vi "Module_ENG_SocketServer.vi"(8 "error in (no error)":errorcluster, 9 "Module ID (-1: Do not Address)":i32=-1, 10 "Wait on Module(s) (\"\": none)":string) -> (0 "error out":errorcluster)   [LabVIEW 2019, in "Module_ENG_SocketServer.lvclass"]
doc: "created using\nJSMA Module Template - ENGINE Class 0.2.1.12\nRob Humfeld - Jet Engineering\nCopyright (c) 2020, Jet Engineering"
uses:
  Module_ENG_SocketServer.lvclass
  <userlib>/Jet Engineering/JSMA/Libraries/jModule Class/Typedefs/jModule_TimerConfig STYP.ctl
  <userlib>/Jet Engineering/JSMA/Libraries/jModule Class/Typedefs/jModule_TimerType STYP.ctl
  Private/Module_ENG_SocketServer_jMsgTxList STYP.ctl
  <userlib>/Jet Engineering/JSMA/Libraries/jMsg_CORE/jMsg_JSMA_ModuleOnline/jMsg_JSMA_ModuleOnline.lvclass
  C:/Program Files/National Instruments/LabVIEW 2019/user.lib/Jet Engineering/JSMA/Libraries/jMsg Class/jMsg.lvclass
  Private/Module_ENG_SocketServer_jMsgRxList STYP.ctl
  <userlib>/Jet Engineering/JSMA/Libraries/jMsg_CORE/jMsg_JSMA_ApplicationShutdown/jMsg_JSMA_ApplicationShutdown.lvclass
  C:/Program Files/National Instruments/LabVIEW 2019/user.lib/Jet Engineering/JSMA/Libraries/jModule Class/jModule.lvclass
  Private/Module_ENG_SocketServer_LocalData STYP.ctl
  Private/Module_ENG_SocketServer_EngineStatus STYP.ctl
  <userlib>/Jet Engineering/JET_QSM/Code/Private/JET_QSM_InvalidOption STYP.ctl
  <userlib>/Jet Engineering/JSMA/Libraries/jModule Class/jModule.lvclass/jModule.ctl
  Module_ENG_SocketServer.lvclass/Module_ENG_SocketServer.ctl
  <userlib>/Jet Engineering/JET_QSM/Code/Private/JET_QSM - Add State [String API].vi
  <userlib>/Jet Engineering/JSMA/Libraries/jModule Class/Read Timeout Configuration.vi
  <userlib>/Jet Engineering/JET_QSM/Code/Private/JET_QSM - Add State to Front [String API].vi
  <vilib>/Utility/error.llb/Trim Whitespace.vi
  <vilib>/Utility/error.llb/Error Cluster From Error Code.vi
  <userlib>/Jet Engineering/JSMA/Libraries/jModule Class/jModule.lvclass
panel:
  out "Timer Configuration":T1 {"Expiration Time" format="%<%.3X>T"}
  out "jModule Name":string
  out "iter":i32
  out "Latency, sec.":dbl
  out "RxTime":timestamp format="%<%H:%M:%S%3u>T"
  out "Last Rx Message":string
  out "Recent states before Error (with tick counts)":string
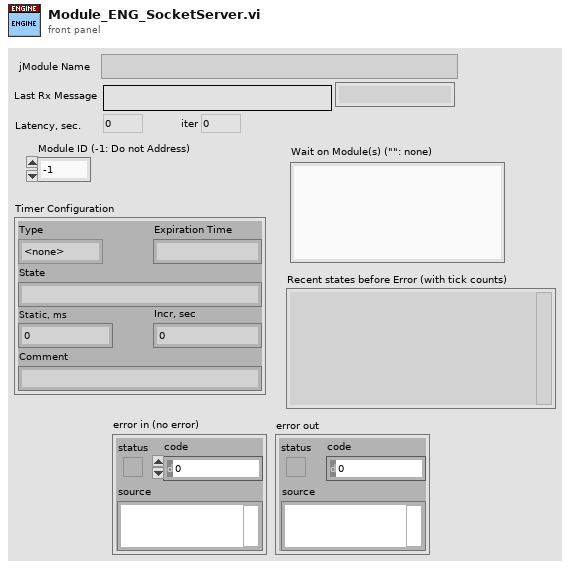
[diagram p1: front panel]
types:
  T1 = typedef "JSMA API.lvlib/jModule.lvclass/jModule_TimerConfig STYP.ctl" = cluster{"Type":T2, "Expiration Time":timestamp, "State":string, "Static, ms":i32, "Incr, sec":dbl, "Comment":string}
  T2 = typedef "JSMA API.lvlib/jModule.lvclass/jModule_TimerType STYP.ctl" = enum16{"<none>", "Static", "Countdown", "Periodic"}
  T3 = typedef "JET_QSM_InvalidOption STYP.ctl" = enum16{"Ignore", "Dialog", "Error"}
  T4 = typedef "Module_ENG_SocketServer.lvclass/Module_ENG_SocketServer_LocalData STYP.ctl" = cluster{"VI":cluster{"error":errorcluster, "isExiting?":bool}, "EngineStatus":T5}
  T5 = typedef "Module_ENG_SocketServer.lvclass/Module_ENG_SocketServer_EngineStatus STYP.ctl" = cluster{"<placeholder>":bool}
  T6 = typedef "Module_ENG_SocketServer.lvclass/Module_ENG_SocketServer_jMsgRxList STYP.ctl" = cluster{"<placeholder>":refnum<class "jMsg_JSMA_ApplicationShutdown.lvclass">}
  T7 = typedef "Module_ENG_SocketServer.lvclass/Module_ENG_SocketServer_jMsgTxList STYP.ctl" = cluster{"<placeholder>":refnum<class "jMsg_JSMA_ModuleOnline.lvclass">}
  T8 = typedef "JET_QSM_Refnum STYP.ctl" = cluster{"state":cluster{"queue":refnum<queue>, "idle":string, "error":string, "STOP":string}, "debug":cluster{"enabled?":bool, "queue":refnum<queue>}, "Invalid.option":T3, "QSM.Name":string}
  T9 = typedef "JET_QSM_Element STYP.ctl" = cluster{"state":string, "data":variant, "comment":string}
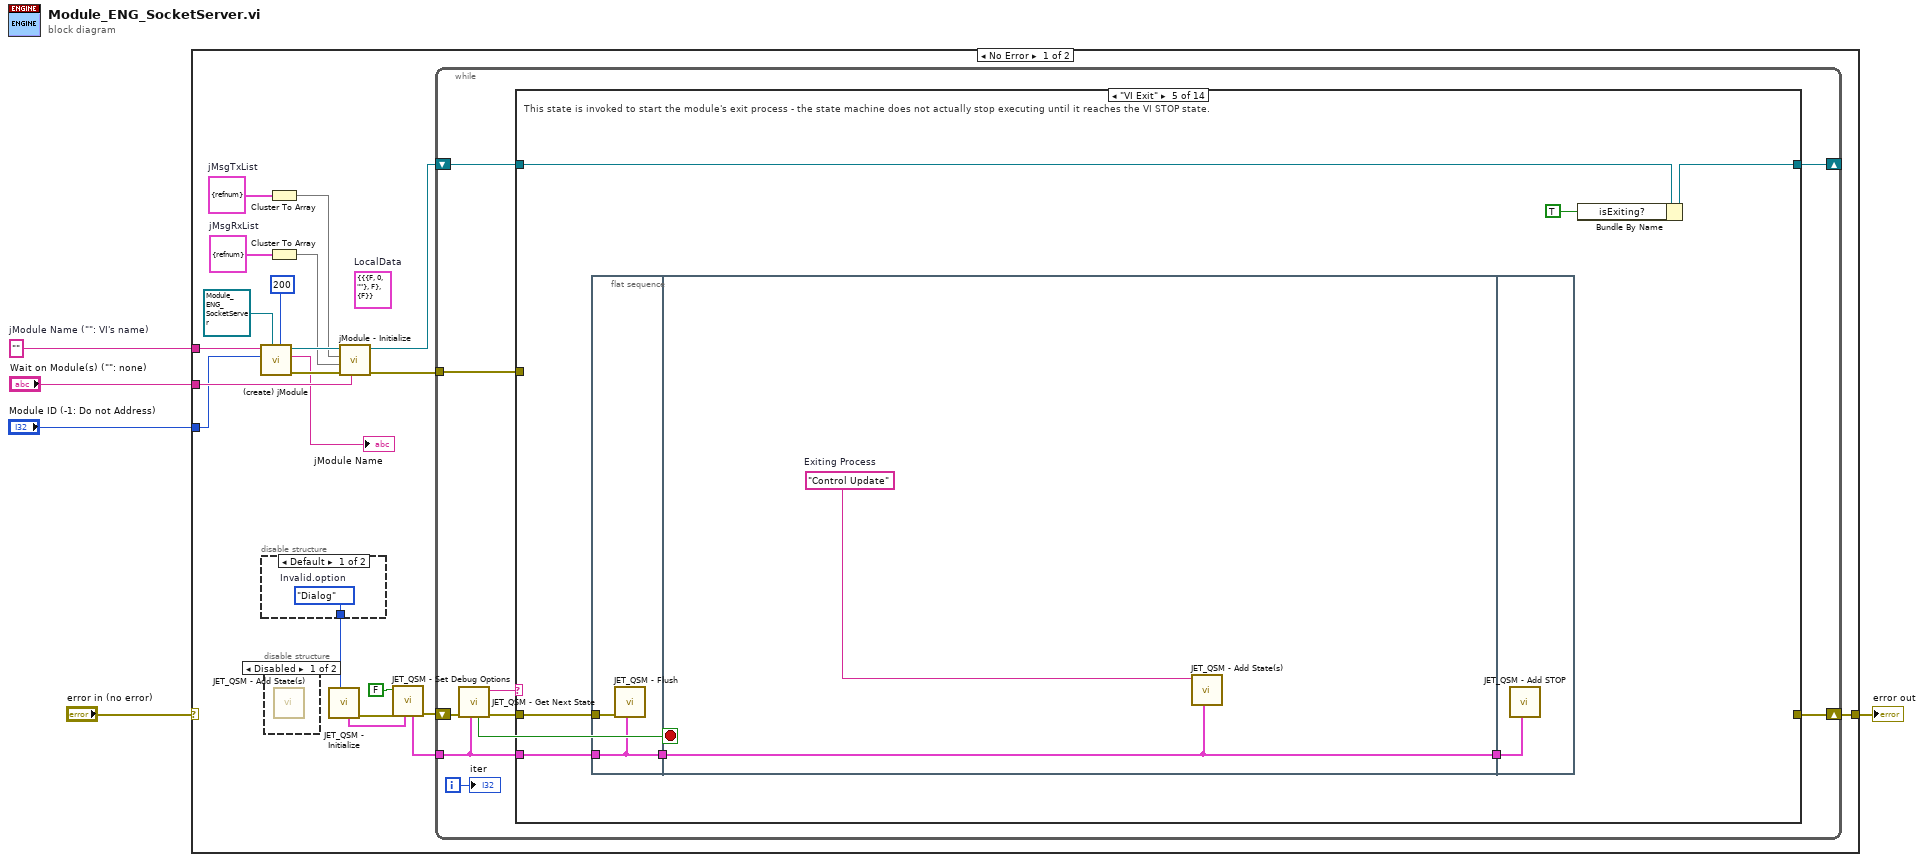
[diagram p0: block diagram]
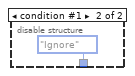
[diagram p3: hidden frame]
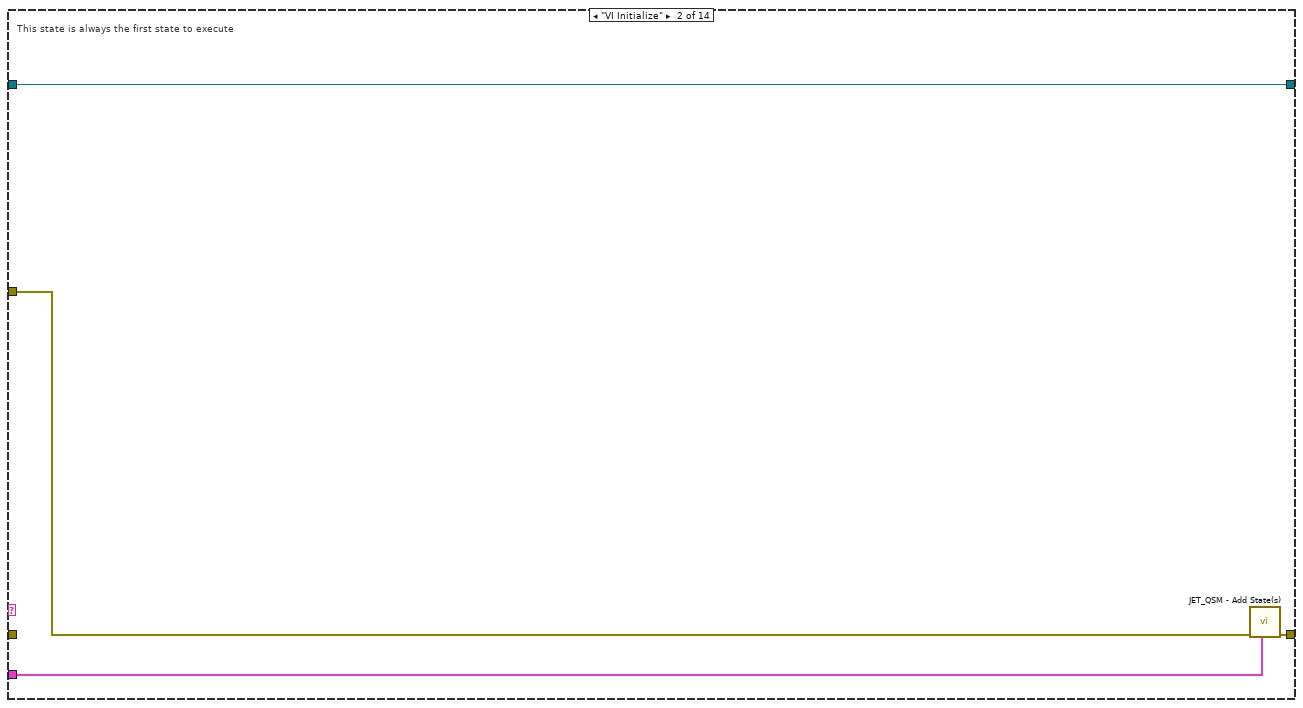
[diagram p5: hidden frame]
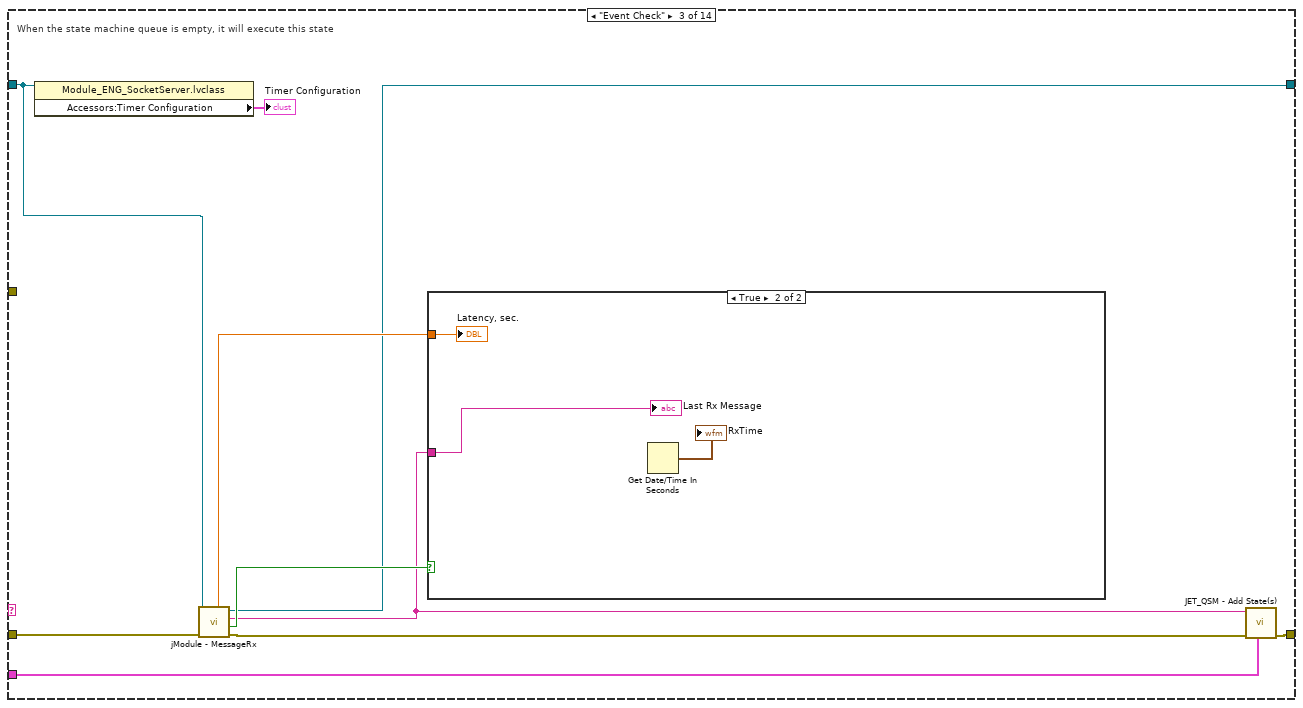
[diagram p6: hidden frame]
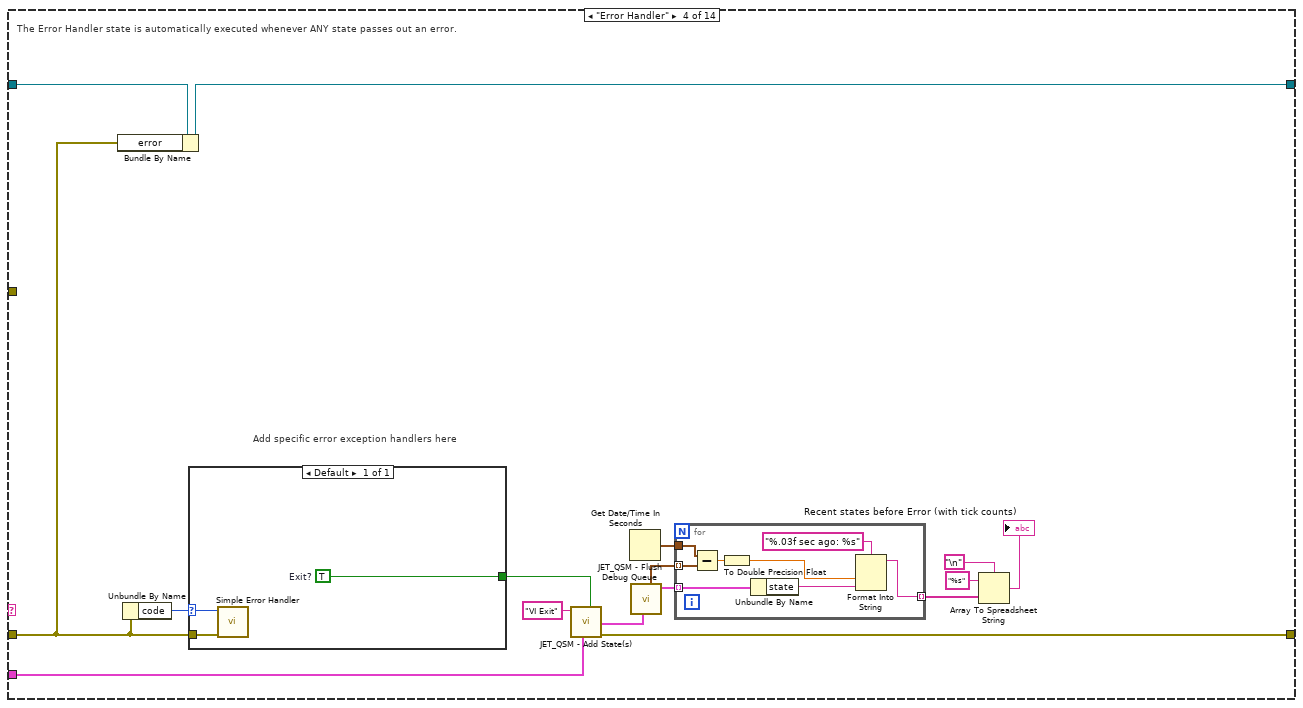
[diagram p8: hidden frame]
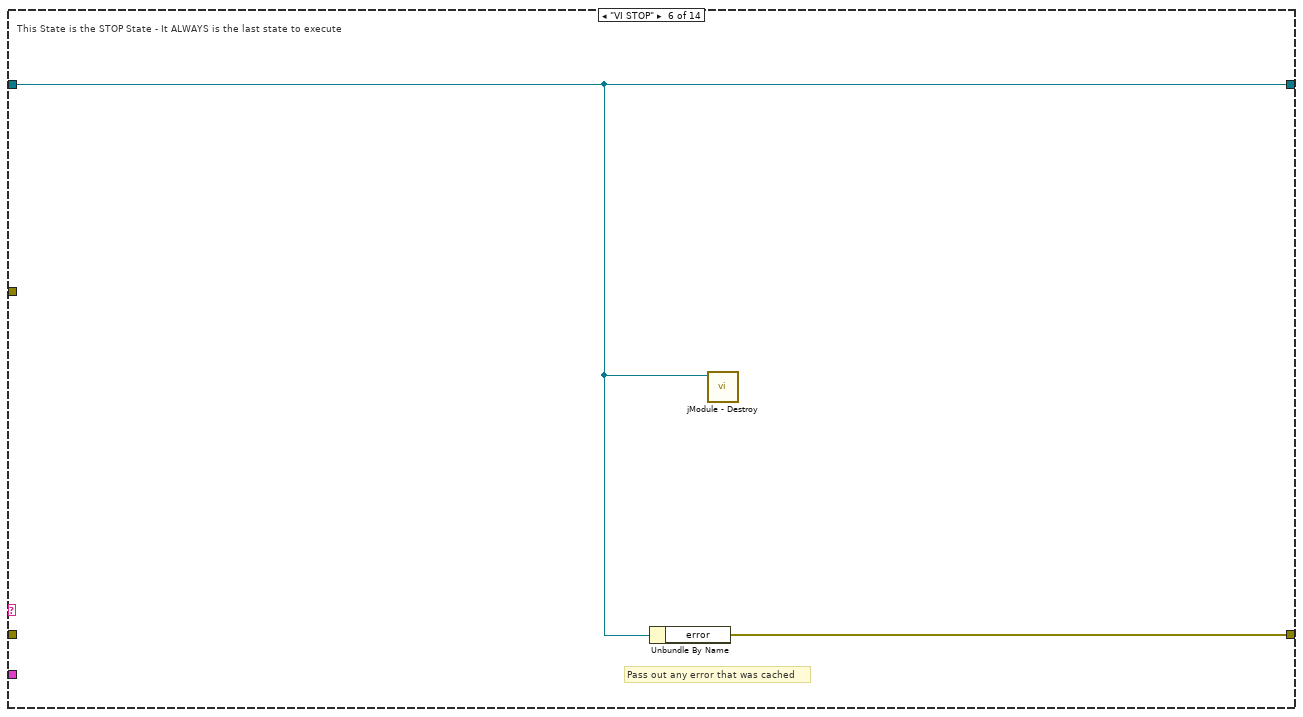
[diagram p9: hidden frame]
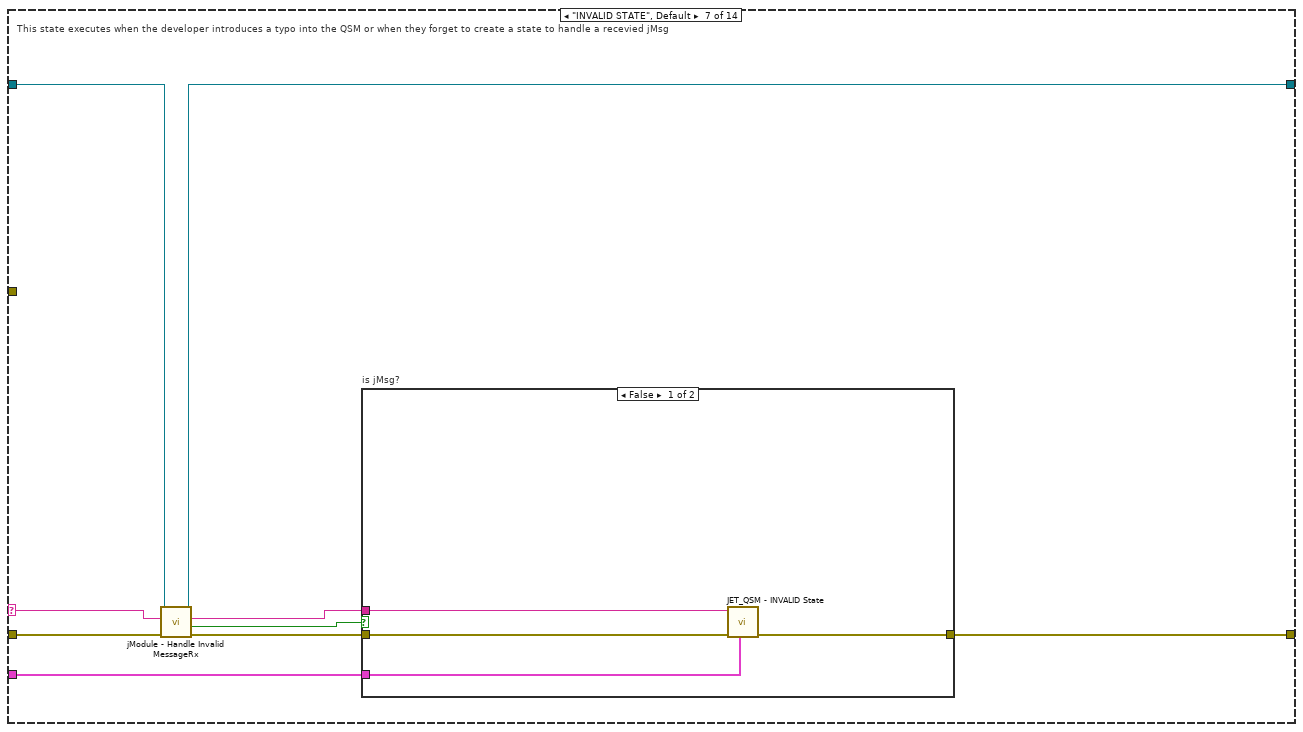
[diagram p10: hidden frame]
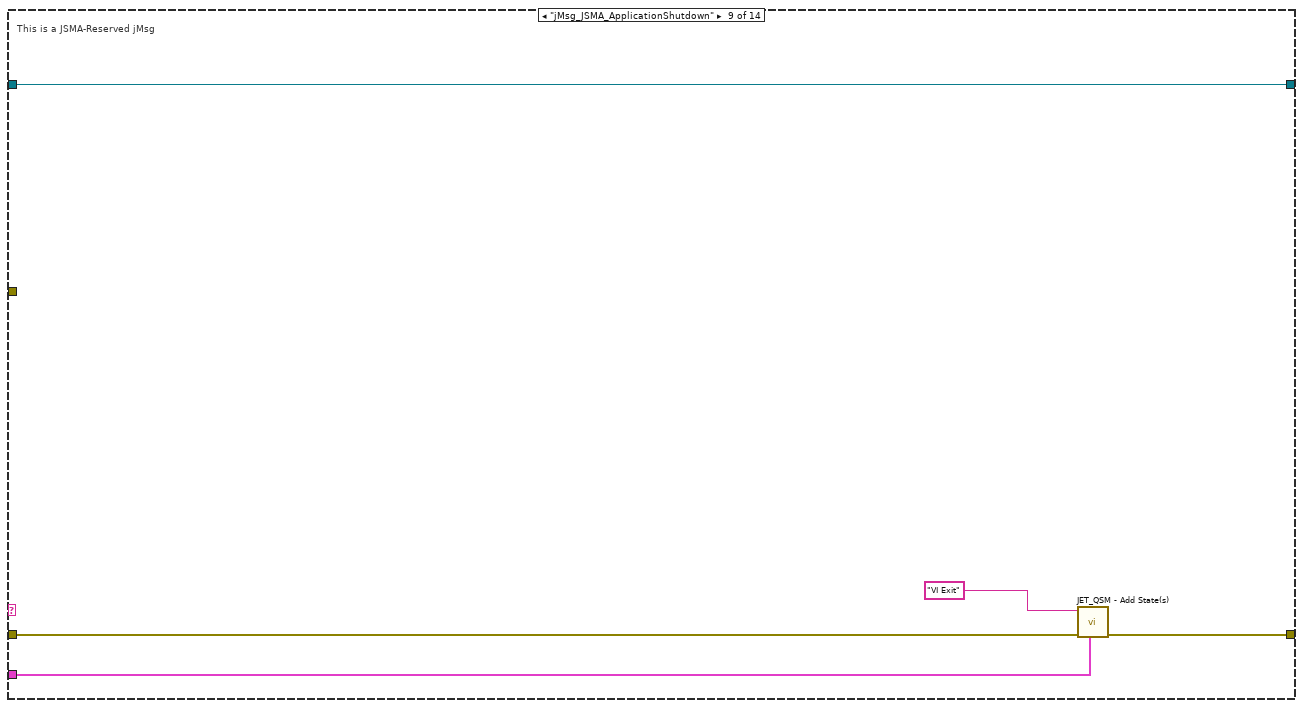
[diagram p13: hidden frame]
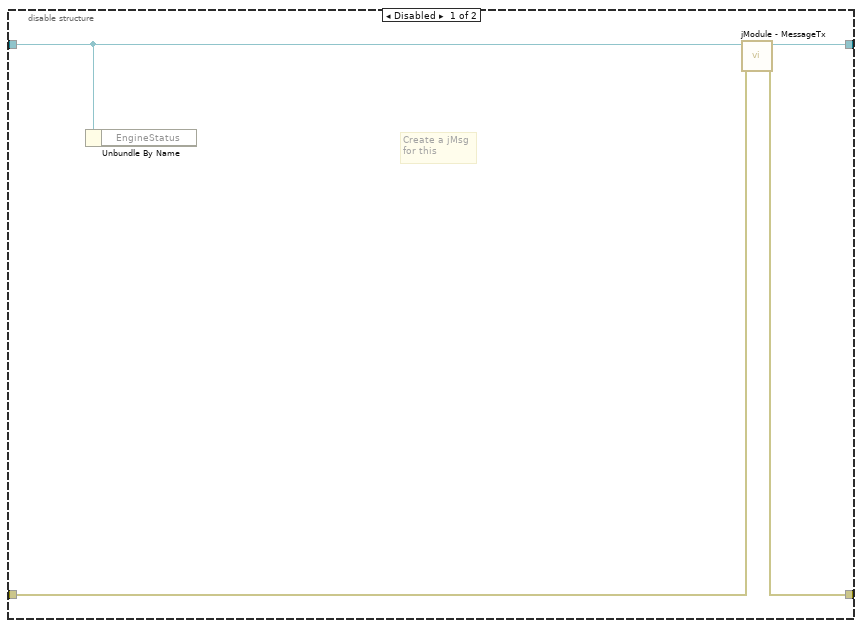
[diagram p16: hidden frame]
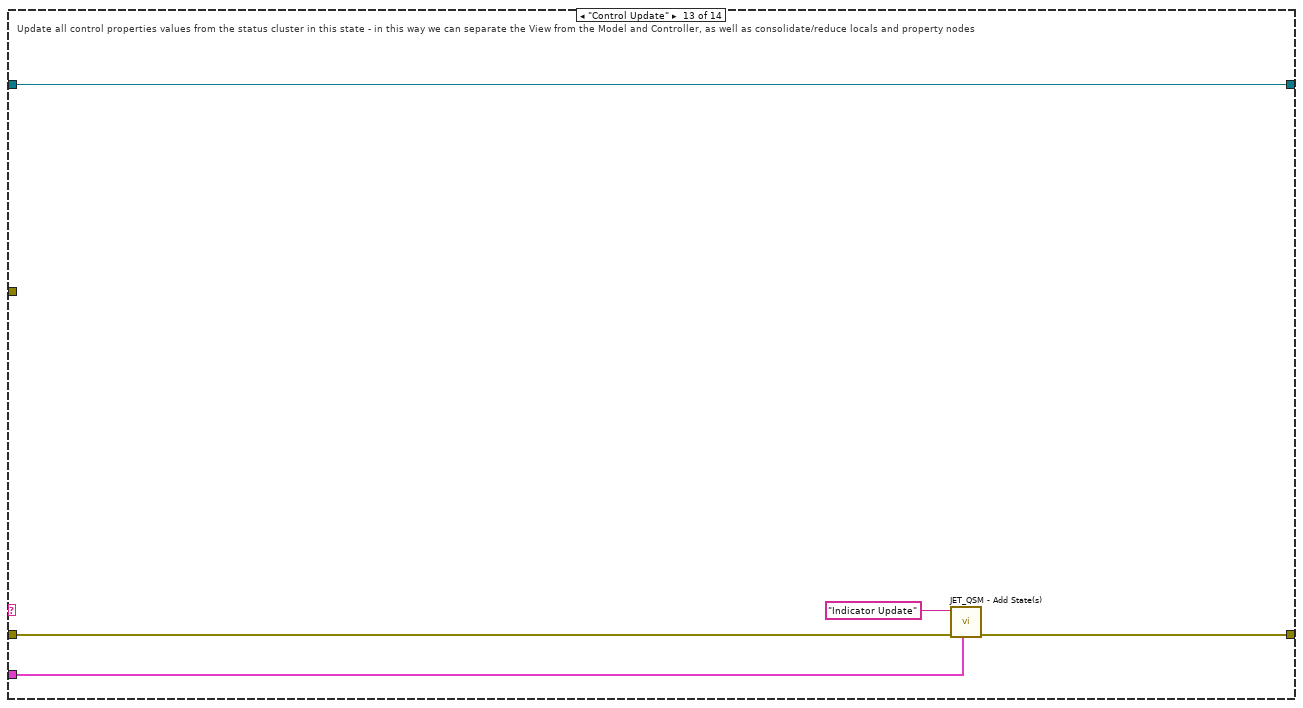
[diagram p18: hidden frame]
diagram:
  w3 = ""  # jModule Name ("": VI's name)
  n1 = case shown="No Error" "error in (no error)" {
    selector: "error in (no error)" -> [_ w140]
    tunnel: [w9 w140] -> w5
    tunnel: "Wait on Module(s) (\"\": none)" -> [w17 _]
    tunnel: w3 -> [w16 _]
    tunnel: "Module ID (-1: Do not Address)" -> [w8 _]
    frame No Error {
      (unwired) T4 {"VI"={"error"={"status"=FALSE, "code"=0, "source"=""}, "isExiting?"=FALSE}, "EngineStatus"={"<placeholder>"=FALSE}}  # LocalData
      w14 = T6 {"<placeholder>"=refnum}  # jMsgRxList
      w15 = T7 {"<placeholder>"=refnum}  # jMsgTxList
      n2 = call <userlib>:"(create) jModule.vi"("Max Queue size (50)"=200, "jModule Child class"=refnum<class "Module_ENG_SocketServer.lvclass"> refnum ("jModule Template_ENGINEClass.lvclass"), "Module ID (-1: Do Not Address)"=w8, "jModule Name (\"\": use calling VI's name)"=w16) -> ("error out"=w19:errorcluster, "jModule Name"=→"jModule Name":string, "jModule"=w22:refnum<class "Module_ENG_SocketServer.lvclass">)  [unwired: 4 in, 1 out]
      n3 = disable-structure shown="Default" {
        disable-tunnel: [w27 JET_QSM_InvalidOption_STYP."Ignore" ("Invalid.option (Dialog)")] -> w18
        frame condition #0 (active) {
          w27 = JET_QSM_InvalidOption_STYP."Dialog"  # Invalid.option
        }
        frame condition #1 {
        }
      }
      n4 = disable-structure shown="Disabled" {
        frame Disabled {
          n5 = call-poly <userlib>:"JET_QSM - Add State(s).vi"() -> ()  [unwired: 11 in, 1 out]
        }
        frame Enabled {
        }
      }
      n6 = Cluster To Array(cluster=w15) -> (array=w21:refnum<class "jMsg_JSMA_ModuleOnline.lvclass">[])
      n7 = Cluster To Array(cluster=w14) -> (array=w20:refnum<class "jMsg_JSMA_ApplicationShutdown.lvclass">[])
      n8 = call <userlib>:"JET_QSM - Initialize.vi"("invalid state action (Dialog)"=w18) -> ("error out"=w23:errorcluster, "Jet_QSM refnum"=w25:T8)  [unwired: 9 in]
      n9 = call-dynamic "jModule - Initialize.vi"("Wait on Module(s) (\"\": none)"=w17, "error in (no error)"=w19, "jMsgRxList"=w20, "jMsgTxList"=w21, "jModule"=w22) -> ("error out"=w11:errorcluster, "jModule"=w10:refnum<class "Module_ENG_SocketServer.lvclass">)  [unwired: 5 in]
      n10 = call <userlib>:"JET_QSM - Set Debug Options.vi"("Jet_QSM refnum"=w25, "error in (no error)"=w23, "debug.enabled? (F)"=FALSE) -> ("error out"=w12:errorcluster, "Jet_QSM ref"=w24:T8)  [unwired: 7 in]
      n11 = while {
        tunnel: w24 -> [w29]
        shift-right: [w33] -> _
        shift-left: w10 -> [w34]
        shift-right: [w32] -> w9
        shift-left: w12 -> [w38]
        tunnel: w11 -> [w30]
        i -> [w31]
        stop <- w35 stop-if-true
        n12 = call <userlib>:"JET_QSM - Get Next State.vi"("Jet_QSM refnum"=w29, "error in (no error)"=w38) -> ("error out"=w37:errorcluster, "state"=w36:string, "Stop Loop?"=w35:bool)  [unwired: 5 in, 2 out]
        n13 = case shown="\"VI Exit\"" w36 {
          selector: w36 -> [_ _ _ _ _ _ w102 _ _ _ _ _ _ _]
          tunnel: w37 -> [w39 _ w52 w62 w90 _ w103 w112 w114 w119 w123 w131 w133 w138]
          tunnel: w34 -> [w40 w42 w48 w59 w85 w97 w99 w113 w115 w120 w121 w132 w134 w139]
          tunnel: [w40 w42 w46 w58 w84 w97 w98 w113 w115 w120 w124 w132 w134 w139] -> w33
          tunnel: [w39 w44 w53 w65 _ w96 w101 w112 w117 w119 w122 w131 w136 w138] -> w32
          tunnel: w30 -> [_ w41 _ _ _ _ _ _ _ _ _ _ _ _]
          tunnel: w29 -> [_ w43 w54 w64 w89 _ w100 _ w118 _ _ _ w137 _]
          frame "------ Standard States ------" {
            # "Standard States are required states for a JET_QSM State Machine\n\nTheir names may be changed; use the Initialize function to specify the new names"
            # "This is a section header; the state is never expected to execute"
          }
          frame "VI Initialize" {
            # "This state is always the first state to execute"
            n14 = call-poly <userlib>:"JET_QSM - Add State(s).vi"("Jet_QSM refnum"=w43, "error in (no error)"=w41) -> ("error out"=w44:errorcluster)  [unwired: 9 in]
          }
          frame "Event Check" {
            # "When the state machine queue is empty, it will execute this state"
            n15 = property class="Module_ENG_SocketServer.lvclass"(reference=w48) -> ("Accessors:Timer Configuration"=→"Timer Configuration":T1)  [unwired: 1 in, 2 out]
            n16 = call-dynamic "jModule - MessageRx.vi"("error in (no error)"=w52, "jModule"=w48) -> ("error out"=w47:errorcluster, "MsgRx?"=w51:bool, "QSMState"=w49:string, "jModule"=w46:refnum<class "Module_ENG_SocketServer.lvclass">, "Latency, sec."=w50:dbl)  [unwired: 4 in, 1 out]
            n17 = case shown="True" w51 {
              tunnel: w49 -> [_ w56]
              tunnel: w50 -> [_ w57]
              frame False {
              }
              frame True {
                n18 = Get Date/Time In Seconds() -> (seconds since 1Jan1904=→"RxTime":timestamp)
                "Last Rx Message" <- w56
                "Latency, sec." <- w57
              }
            }
            n19 = call-poly <userlib>:"JET_QSM - Add State(s).vi"("Jet_QSM refnum"=w54, "error in (no error)"=w47, "state(s)"=w49) -> ("error out"=w53:errorcluster)  [unwired: 8 in]
          }
          frame "Error Handler" {
            # "Add specific error exception handlers here"
            # "The Error Handler state is automatically executed whenever ANY state passes out an error."
            n20 = Bundle By Name(cluster=w59, "error"=w62) -> (w58:refnum<class "Module_ENG_SocketServer.lvclass">)
            n21 = Unbundle By Name(w62) -> ("code"=w60:i32)
            n22 = case shown="Default" w60 {
              selector: w60 -> [w74]
              tunnel: [w75] -> w61
              tunnel: w62 -> [w73]
              frame Default {
                w75 = TRUE  # Exit?
                n23 = call <vilib>:"Simple Error Handler.vi"("error code (no error:0)"=w74, "error in (no error)"=w73) -> ()  [unwired: 3 in, 5 out]
              }
            }
            n24 = call-poly <userlib>:"JET_QSM - Add State(s).vi"("act? (T)"=w61, "Jet_QSM refnum"=w64, "state(s)"="VI Exit") -> ("error out"=w65:errorcluster)  [unwired: 8 in]
            n25 = Get Date/Time In Seconds() -> (seconds since 1Jan1904=w68:timestamp)
            n26 = call <userlib>:"JET_QSM - Flush Debug Queue.vi"("Jet_QSM refnum"=w64) -> ("QSM Elements"=w66:T9[], "Timestamps"=w67:timestamp[])  [unwired: 8 in, 1 out]
            n27 = for {
              tunnel: w66 -> [w83] mode=indexing
              tunnel: [w81] -> w70 mode=indexing
              tunnel: w68 -> [w78]
              tunnel: w67 -> [w79] mode=indexing
              n28 = Subtract(x=w78, y=w79) -> (x-y=w77:dbl)
              n29 = To Double Precision Float(number=w77) -> (double precision float=w76:dbl)
              n30 = Unbundle By Name(w83) -> ("state"=w82:string)
              n31 = Format Into String(format string="%.03f sec ago: %s", w76, w82) -> (resulting string=w81:string)  [unwired: 2 in, 1 out]
            }
            n32 = Array To Spreadsheet String(delimiter (Tab)="\n", array=w70, 3:"%s" ("format string")) -> (spreadsheet string=→"Recent states before Error (with tick counts)":string)
          }
          frame "VI Exit" {
            # "This state is invoked to start the module's exit process - the state machine does not actually stop executing until it reaches the VI STOP state."
            n33 = flat-sequence {
              tunnel: w90 -> [w92]
              tunnel: w89 -> [w91]
              tunnel: [w91] -> w88
              tunnel: w88 -> [w94]
              tunnel: [w94] -> w87
              tunnel: w87 -> [w95]
              frame #0 {
                n34 = call <userlib>:"JET_QSM - Flush.vi"("Jet_QSM ref"=w91, "error in (no error)"=w92) -> ()  [unwired: 8 in, 2 out]
              }
              frame #1 {
                w93 = "Control Update"  # Exiting Process
                n35 = call-poly <userlib>:"JET_QSM - Add State(s).vi"("Jet_QSM refnum"=w94, "state(s)"=w93) -> ()  [unwired: 9 in, 1 out]
              }
              frame #2 {
                n36 = call <userlib>:"JET_QSM - Add STOP.vi"("Jet_QSM refnum"=w95) -> ()  [unwired: 10 in, 1 out]
              }
            }
            n37 = Bundle By Name(cluster=w85, "isExiting?"=TRUE ("VI.isExiting?")) -> (w84:refnum<class "Module_ENG_SocketServer.lvclass">)
          }
          frame "VI STOP" {
            # "Pass out any error that was cached"
            # "This State is the STOP State - It ALWAYS is the last state to execute"
            n38 = Unbundle By Name(w97) -> ("error"=w96:errorcluster)
            n39 = call-dynamic "jModule - Destroy.vi"("jModule"=w97) -> ()  [unwired: 10 in, 1 out]
          }
          frame "INVALID STATE", Default {
            # "This state executes when the developer introduces a typo into the QSM or when they forget to create a state to handle a recevied jMsg"
            n40 = call-dynamic "jModule - Handle Invalid MessageRx.vi"("error in (no error)"=w103, "Invalid State"=w102, "jModule"=w99) -> ("error out"=w106:errorcluster, "is jMsg State?"=w104:bool, "Invalid State"=w105:string, "jModule"=w98:refnum<class "Module_ENG_SocketServer.lvclass">)  [unwired: 5 in]
            n41 = case "is jMsg?" shown="False" w104 {
              tunnel: w100 -> [w108 _]
              tunnel: [w107 w111] -> w101
              tunnel: w106 -> [w109 w111]
              tunnel: w105 -> [w110 _]
              frame False {
                n42 = call <userlib>:"JET_QSM - INVALID State.vi"("Jet_QSM refnum"=w108, "error in (no error)"=w109, "state"=w110) -> ("error out"=w107:errorcluster)  [unwired: 8 in]
              }
              frame True {
              }
            }
          }
          frame "------ jMsg  ------" {
            # "This is a section header; the state is never expected to execute"
          }
          frame "jMsg_JSMA_ApplicationShutdown" {
            # "This is a JSMA-Reserved jMsg"
            n43 = call-poly <userlib>:"JET_QSM - Add State(s).vi"("Jet_QSM refnum"=w118, "error in (no error)"=w114, "state(s)"="VI Exit") -> ("error out"=w117:errorcluster)  [unwired: 8 in]
          }
          frame "------ Actions  ------" {
            # "This is a section header; the state is never expected to execute"
          }
          frame "Send: Status Update" {
            # "This is how your engine broadcasts its status to the application"
            n44 = disable-structure shown="Enabled" {
              disable-tunnel: [w127 w130] -> w124
              disable-tunnel: w123 -> [w126 w129]
              disable-tunnel: [w125 w129] -> w122
              disable-tunnel: w121 -> [w128 w130]
              frame Disabled {
                # "Create a jMsg\nfor this"
                n45 = Unbundle By Name(w128) -> ()  [unwired: 1 out]
                n46 = call <userlib>:"jModule - MessageTx.vi"("error in (no error)"=w126, "jModule"=w128) -> ("error out"=w125:errorcluster, "jModule"=w127:refnum<class "Module_ENG_SocketServer.lvclass">)  [unwired: 6 in, 2 out]
              }
              frame Enabled {
              }
            }
          }
          frame "------ Window and Panel Control ------" {
            # "This is a section header; the state is never expected to execute"
          }
          frame "Control Update" {
            # "Update all control properties values from the status cluster in this state - in this way we can separate the View from the Model and Controller, as well as consolidate/reduce locals and property nodes"
            n47 = call-poly <userlib>:"JET_QSM - Add State(s).vi"("Jet_QSM refnum"=w137, "error in (no error)"=w133, "state(s)"="Indicator Update") -> ("error out"=w136:errorcluster)  [unwired: 8 in]
          }
          frame "Indicator Update" {
            # "Update all indicator properties and values from the status cluster in this state - in this way we can separate the View from the Model and Controller, as well as consolidate/reduce property nodes"
          }
        }
        "iter" <- w31
      }
    }
    frame Error {
    }
  }
  "error out" <- w5
